vi "motorpractice.vi"() -> ()   [LabVIEW 2014]
uses:
  <vilib>/Motion/FlexMotion/CustomControls/CustomControls.llb/AxisOrVectorSpace To Configure.flx
  <vilib>/Motion/FlexMotion/FunctionsVIs/StartStopMotion.llb/Start Motion (8 axes).flx
  <vilib>/Motion/FlexMotion/FunctionsVIs/Trajectory.llb/Check Move Complete Status (8 axes).flx
  <vilib>/Motion/FlexMotion/FunctionsVIs/StartStopMotion.llb/Stop Motion (8 axes).flx
panel:
  in  "Velocity (10000)":i32=10000 min=-20000000 max=20000000
  in  "Target Position (0)":i32
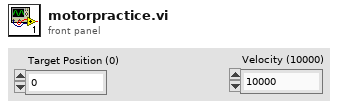
[diagram p1: front panel]
types:
  T1 = typedef "Board Id" = u8
  T2 = enum16{"Absolute Position", "Relative Position", "Velocity", "Relative to Cap Pos", "Modulus Position", "Absolute Contouring", "Relative Contouring"}
  T3 = typedef "AxisOrVectorSpace To Configure.flx" = u16
  T4 = typedef "Resource Out (Enum).flx" = u16
  T5 = typedef "Bd Id Out" = u8
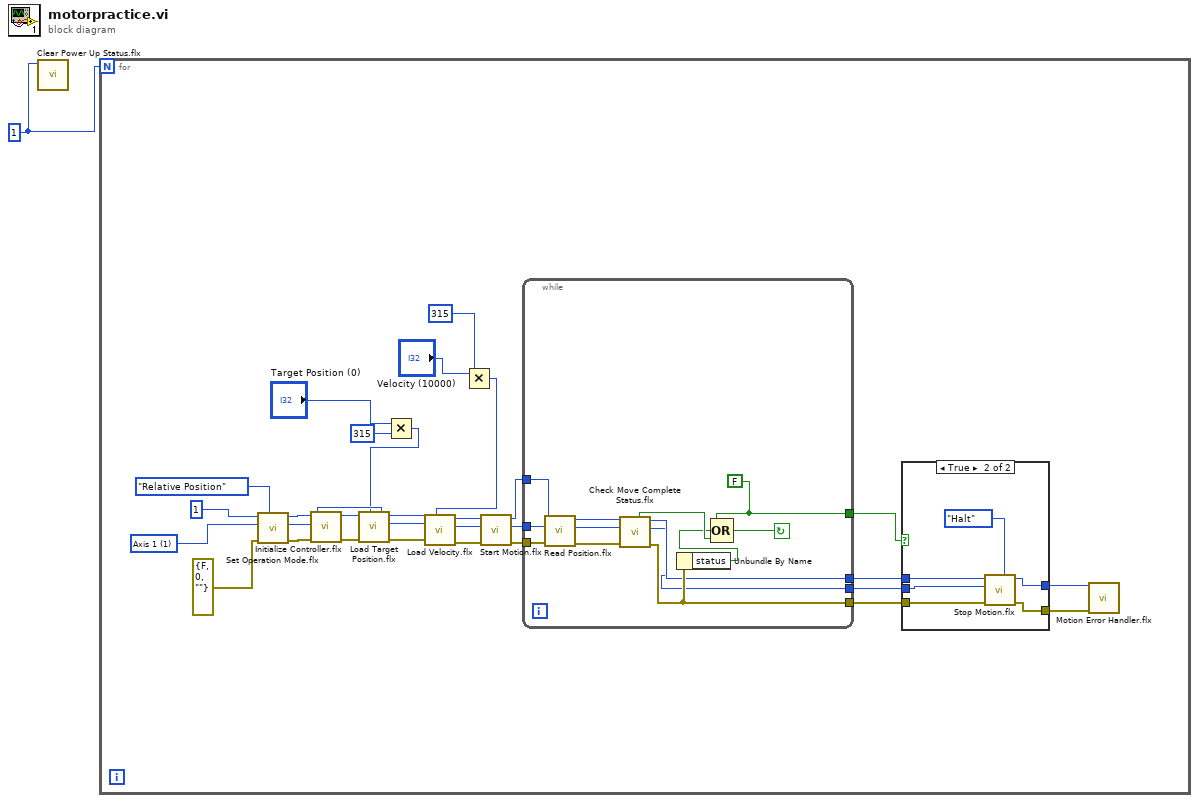
[diagram p0: block diagram]
diagram:
  w1 = T1 1 ("Board ID")
  n1 = call <vilib>:"Clear Power Up Status.flx"("Board ID"=w1) -> ()  [unwired: 6 in, 2 out]
  n2 = for {
    N: w1 -> [_]
    w29 = T3 1 items=["Axis 1"=1, "Axis 2"=2, "Axis 3"=3, "Axis 4"=4, "Axis 5"=5, "Axis 6"=6, "Axis 7"=7, "Axis 8"=8, "Vector Space 1"=17, "Vector Space 2"=18, "Vector Space 3"=19, "Vector Space 4"=20] ("Axis or Vector Space")
    n3 = call <vilib>:"Set Operation Mode.flx"("Position Mode (Absolute)"=T2."Relative Position", "error in (no error)"=errorcluster {"status"=FALSE, "code"=0, "source"=""} ("error constant"), "Axis or Vector Space"=w29, "Board ID"=T1 1) -> ("error out"=w27:errorcluster, "Resource Output"=w26:T4, "Bd ID Out"=w25:T5)  [unwired: 2 in]
    n4 = call <vilib>:"Initialize Controller.flx"("error in (no error)"=w27, "Board ID"=w25) -> ("error out"=w20:errorcluster, "Bd ID Out"=w24:T5)  [unwired: 6 in]
    n5 = Multiply(x="Target Position (0)", y=315) -> (x*y=w5:i32)
    n6 = call <vilib>:"Load Target Position.flx"("Target Position (0)"=w5, "error in (no error)"=w20, "Axis"=w26, "Board ID"=w24) -> ("error out"=w21:errorcluster, "Resource Output"=w22:T4, "Bd ID Out"=w23:T5)  [unwired: 3 in]
    n7 = Multiply(x="Velocity (10000)", y=315) -> (x*y=w2:i32)
    n8 = call <vilib>:"Load Velocity.flx"("Velocity (10000)"=w2, "error in (no error)"=w21, "Axis or Vector Space"=w22, "Board ID"=w23) -> ("error out"=w17:errorcluster, "Resource Output"=w18:T4, "Bd ID Out"=w19:T5)  [unwired: 3 in]
    n9 = call-poly <vilib>:"Start Motion.flx"("error in (no error)"=w17, "Axis or Vector Space"=w18, "Board ID"=w19) -> ("error out"=w14:errorcluster, "Resource Output"=w15:T4, "Bd ID Out"=w16:T5)  [unwired: 3 in]
    n10 = while {
      tunnel: w16 -> [w52]
      tunnel: w15 -> [w51]
      tunnel: w14 -> [w50]
      tunnel: [w44] -> w13
      tunnel: [w43] -> w12
      tunnel: [w41] -> w11
      tunnel: [w40] -> w10
      stop <- w45 continue-if-true
      w44 = FALSE
      n11 = call <vilib>:"Read Position.flx"("error in (no error)"=w50, "Axis"=w51, "Board ID"=w52) -> ("error out"=w47:errorcluster, "Resource Output"=w48:T4, "Bd ID Out"=w49:T5)  [unwired: 3 in, 1 out]
      n12 = call-poly <vilib>:"Check Move Complete Status.flx"("error in (no error)"=w47, "Axis or Vector Space"=w48, "Board ID"=w49) -> ("error out"=w43:errorcluster, "Resource Output"=w40:T4, "Bd ID Out"=w41:T5, "Move Complete"=w46:bool)  [unwired: 3 in]
      n13 = Unbundle By Name(w43) -> ("status"=w42:bool)
      n14 = Compound Arithmetic op=OR(w44, w42, w46) -> (w45:bool)
    }
    n15 = case shown="True" w13 {
      tunnel: w12 -> [w32 w38]
      tunnel: w11 -> [w33 w37]
      tunnel: w10 -> [_ w36]
      tunnel: [w32 w35] -> w9
      tunnel: [w33 w34] -> w8
      frame False {
      }
      frame True {
        n16 = call-poly <vilib>:"Stop Motion.flx"("Stop Type (Decel)"=enum16{"Decelerate", "Halt", "Kill"}."Halt", "error in (no error)"=w38, "Axis or Vector Space"=w36, "Board ID"=w37) -> ("error out"=w35:errorcluster, "Bd ID Out"=w34:T5)  [unwired: 3 in, 1 out]
      }
    }
    n17 = call <vilib>:"Motion Error Handler.flx"("Board ID"=w8, "error in (no error)"=w9) -> ()  [unwired: 9 in, 5 out]
  }
